vi "UDD Pulse Sequence Generator.vi"(0 "Rabi Frequency":dbl, 1 "No. Instructions":i32, 3 "Array":T1(array[cluster]), 5 "Tau min":dbl, 9 "Tau max":dbl, 11 "Tau step size":dbl, 12 "MW Delay":dbl, 13 "0->+?":bool, 14 "No. Pi Pulses":i32, 15 "Pulse offset":dbl) -> (4 "Pulse Sequence":T1(array[cluster]), 6 "Tau":dbl[](array[numeric]))   [LabVIEW 2012]
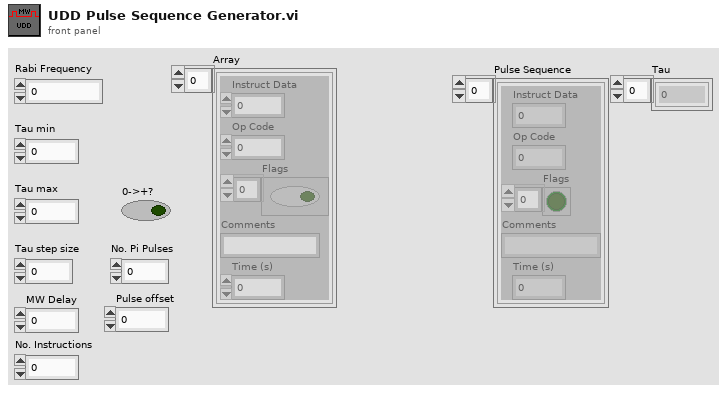
[diagram p1: front panel]
types:
  T1 = cluster{"Instruct Data":i32, "Op Code":i32, "Flags":bool[], "Comments":string, "Time (s)":dbl}[]
  T2 = cluster{"Instruct Data":i32, "Op Code":i32, "Flags":bool[], "Comments":string, "Time (s)":dbl}
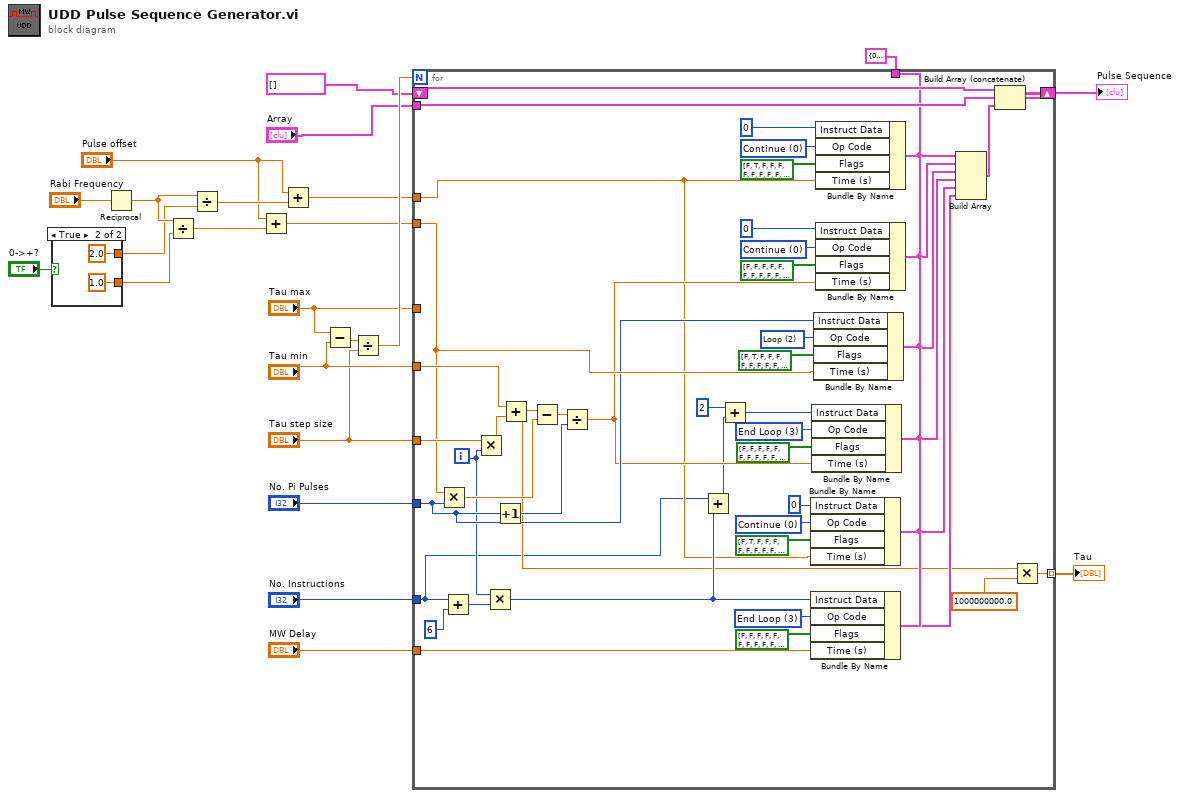
[diagram p0: block diagram]
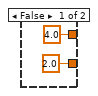
[diagram p2: hidden frame]
diagram:
  n1 = case shown="True" "0->+?" {
    tunnel: [4.0 ("y") 2.0 ("y")] -> w3
    tunnel: [2.0 ("y") 1.0 ("y")] -> w2
    frame False {
    }
    frame True {
    }
  }
  n2 = Reciprocal(x="Rabi Frequency") -> (1/x=w9:dbl)
  n3 = Divide(x=w9, y=w2) -> (x/y=w8:dbl)
  n4 = Divide(x=w9, y=w3) -> (x/y=w20:dbl)
  n5 = Add(x="Pulse offset", y=w8) -> (x+y=w6:dbl)
  n6 = Add(x="Pulse offset", y=w20) -> (x+y=w10:dbl)
  n7 = Subtract(x="Tau max", y="Tau min") -> (x-y=w23:dbl)
  n8 = Divide(x=w23, y="Tau step size") -> (x/y=w22:dbl)
  n9 = for {
    N: w22 -> [_]
    tunnel: w10 -> [w31]
    tunnel: "Tau max" -> [_]
    tunnel: "Tau min" -> [w45]
    tunnel: "Tau step size" -> [w47]
    shift-right: [w72] -> w12
    shift-left: T1 [] -> [w71]
    tunnel: "Array" -> [w70]
    tunnel: T2 {"Instruct Data"=0, "Op Code"=0, "Flags"=[FALSE, FALSE, FALSE, FALSE, FALSE, FALSE, FALSE, FALSE, FALSE, FALSE, FALSE, FALSE, FALSE, FALSE, FALSE, FALSE, FALSE, FALSE, FALSE, FALSE, FALSE, TRUE, TRUE, TRUE], "Comments"="", "Time (s)"=0.01} ("PB Inst 2") -> [w57]
    tunnel: "MW Delay" -> [w41]
    tunnel: [w48] -> w11 mode=indexing
    tunnel: w6 -> [w40]
    tunnel: "No. Pi Pulses" -> [w39]
    tunnel: "No. Instructions" -> [w28]
    i -> [w34]
    w58 = 3 items=["Continue", "Stop", "Loop", "End Loop", "JSR", "RTS", "Branch", "Long Delay", "Wait"] ("Op Code")
    w61 = 0 items=["Continue", "Stop", "Loop", "End Loop", "JSR", "RTS", "Branch", "Long Delay", "Wait"] ("Op Code")
    w63 = 3 items=["Continue", "Stop", "Loop", "End Loop", "JSR", "RTS", "Branch", "Long Delay", "Wait"] ("Op Code")
    w65 = 2 items=["Continue", "Stop", "Loop", "End Loop", "JSR", "RTS", "Branch", "Long Delay", "Wait"] ("Op Code")
    w68 = 0 items=["Continue", "Stop", "Loop", "End Loop", "JSR", "RTS", "Branch", "Long Delay", "Wait"] ("Op Code")
    w74 = 0 items=["Continue", "Stop", "Loop", "End Loop", "JSR", "RTS", "Branch", "Long Delay", "Wait"] ("Op Code")
    n10 = Multiply(x=w40, y=w39) -> (x*y=w43:dbl)
    n11 = Add(x=w28, y=6) -> (x+y=w35:i32)
    n12 = Multiply(x=w47, y=w34) -> (x*y=w46:dbl)
    n13 = Multiply(x=w34, y=w35) -> (x*y=w33:i32)
    n14 = Increment(x=w39) -> (x+1=w42:i32)
    n15 = Add(x=w45, y=w46) -> (x+y=w30:dbl)
    n16 = Subtract(x=w30, y=w43) -> (x-y=w44:dbl)
    n17 = Divide(x=w44, y=w42) -> (x/y=w38:dbl)
    n18 = Add(x=w28, y=w33) -> (x+y=w29:i32)
    n19 = Add(x=2, y=w29) -> (x+y=w32:i32)
    n20 = Bundle By Name(cluster=w57, "Instruct Data"=0, "Op Code"=w61, "Flags"=bool[] [FALSE, TRUE, FALSE, FALSE, FALSE, FALSE, FALSE, FALSE, FALSE, FALSE, FALSE, FALSE, FALSE, FALSE, FALSE, FALSE, FALSE, FALSE, FALSE, FALSE, FALSE, TRUE, TRUE, TRUE], "Time (s)"=w31) -> (w53:T2)
    n21 = Bundle By Name(cluster=w57, "Instruct Data"=w33, "Op Code"=w58, "Flags"=bool[] [FALSE, FALSE, FALSE, FALSE, FALSE, FALSE, FALSE, FALSE, FALSE, FALSE, FALSE, FALSE, FALSE, FALSE, FALSE, FALSE, FALSE, FALSE, FALSE, FALSE, FALSE, TRUE, TRUE, TRUE], "Time (s)"=w41) -> (w54:T2)
    n22 = Bundle By Name(cluster=w57, "Instruct Data"=w32, "Op Code"=w63, "Flags"=bool[] [FALSE, FALSE, FALSE, FALSE, FALSE, FALSE, FALSE, FALSE, FALSE, FALSE, FALSE, FALSE, FALSE, FALSE, FALSE, FALSE, FALSE, FALSE, FALSE, FALSE, FALSE, TRUE, TRUE, TRUE], "Time (s)"=w38) -> (w52:T2)
    n23 = Bundle By Name(cluster=w57, "Instruct Data"=w39, "Op Code"=w65, "Flags"=bool[] [FALSE, TRUE, FALSE, FALSE, FALSE, FALSE, FALSE, FALSE, FALSE, FALSE, FALSE, FALSE, FALSE, FALSE, FALSE, FALSE, FALSE, FALSE, FALSE, FALSE, FALSE, TRUE, TRUE, TRUE], "Time (s)"=w40) -> (w51:T2)
    n24 = Bundle By Name(cluster=w57, "Instruct Data"=0, "Op Code"=w74, "Flags"=bool[] [FALSE, TRUE, FALSE, FALSE, FALSE, FALSE, FALSE, FALSE, FALSE, FALSE, FALSE, FALSE, FALSE, FALSE, FALSE, FALSE, FALSE, FALSE, FALSE, FALSE, FALSE, TRUE, TRUE, TRUE], "Time (s)"=w31) -> (w55:T2)
    n25 = Bundle By Name(cluster=w57, "Instruct Data"=0, "Op Code"=w68, "Flags"=bool[] [FALSE, FALSE, FALSE, FALSE, FALSE, FALSE, FALSE, FALSE, FALSE, FALSE, FALSE, FALSE, FALSE, FALSE, FALSE, FALSE, FALSE, FALSE, FALSE, FALSE, FALSE, TRUE, TRUE, TRUE], "Time (s)"=w38) -> (w50:T2)
    n26 = Build Array(w55, w50, w51, w52, w53, w54) -> (w56:T1)
    n27 = Build Array (concatenate)(w71, w70, w56) -> (w72:T1)
    n28 = Multiply(x=w30, y=1000000000.0) -> (x*y=w48:dbl)
  }
  "Pulse Sequence" <- w12
  "Tau" <- w11
